vi "MEScope_GetDspVer.vi"(8 "error in (no error)":errorcluster) -> (0 "error out":errorcluster, 1 "return type":i32, 3 "szTargBuff":string)   [LabVIEW 2015]
doc: "MEScope_GetDspVer\n\nDescription:\nThis test will return the version number of the DSP code in a string.\nDetail:\nint MEScope_GetDspVer (\nchar *szTargBuff\n);\n\nParameters:\nchar *szTargBuff - Pointer to a character buffer of no larger than 80 bytes. \n\nReturn Values:\nA returned value of 0 indicates success, with the appropriate strings in the buffer. Otherwise, treat the returned value as an error code."
uses:
  ScannerDiagDLL.dll
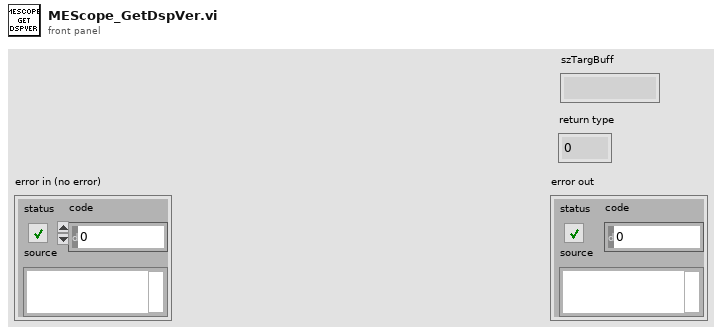
[diagram p1: front panel]
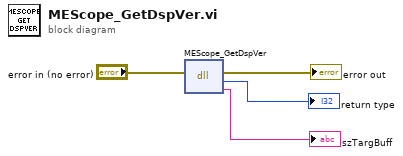
[diagram p0: block diagram]
diagram:
  n1 = dll-call lib="C:/ModisEdge/Scope/Test Sequence/Code Modules/DLL/ScannerDiagDLL.dll" fn="MEScope_GetDspVer"(error in="error in (no error)") -> (error out=→"error out":errorcluster, "return type"=→"return type":i32, "szTargBuff"=→"szTargBuff":string)  [unwired: 3 in, 1 out]
